vi "TCL Select Fragments 1frag1criterium.vi"(0 "event file":path, 1 "fragment":string, 3 "primary key":string, 4 "criterium":T1={"fragment"="", "values"=[], "operator"="is equal to"}, 5 "error in (no error)":errorcluster) -> (6 "fragments out":string[](array[string]), 7 "matches":string[][](array[string]), 8 "error out":errorcluster)   [LabVIEW 2010]
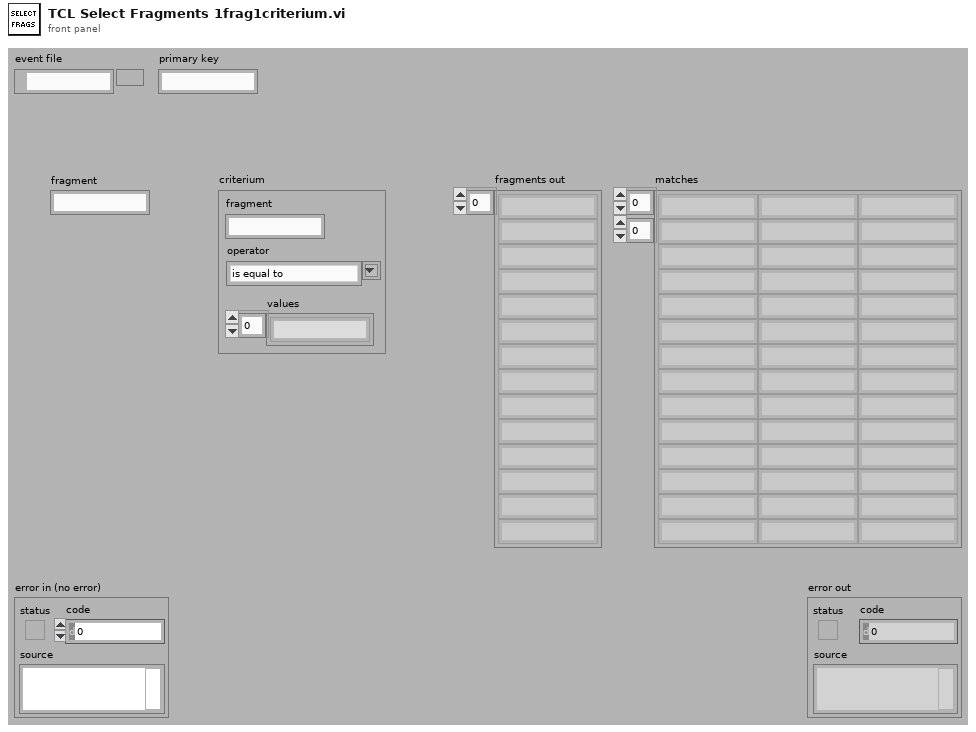
[diagram p1: front panel]
types:
  T1 = cluster{"fragment":string, "values":string[], "operator":string}
  T2 = cluster{"fragment":string, "values":string[], "operator":string}[]
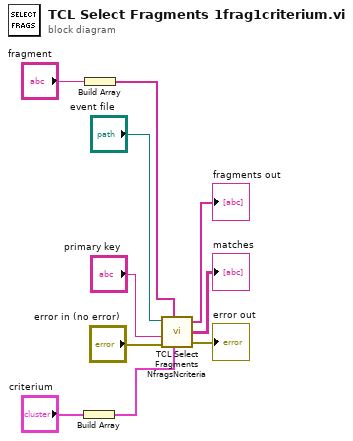
[diagram p0: block diagram]
diagram:
  n1 = Build Array("criterium") -> (w9:T2)
  n2 = Build Array("fragment") -> (w8:string[])
  n3 = call "TCL Select Fragments NfragsNcriteria.vi"("event file"="event file", "fragments"=w8, "primary key"="primary key", "criteria"=w9, "error in (no error)"="error in (no error)") -> ("fragments out"=→"fragments out":string[], "matches"=→"matches":string[][], "error out"=→"error out":errorcluster)  [unwired: 1 in]
